vi "calculate_frequency.vi"(8 "error in (no error)":errorcluster, 10 "array with duplicates removed":string[](array[string]), 11 "String data spreadsheet":string) -> (0 "error out":errorcluster, 1 "Array":i32[](array[numeric]), 2 "Frequency of numbers":string[][](array[string]), 3 "Cluster":cluster{i32[], i32[]})   [LabVIEW 2020]
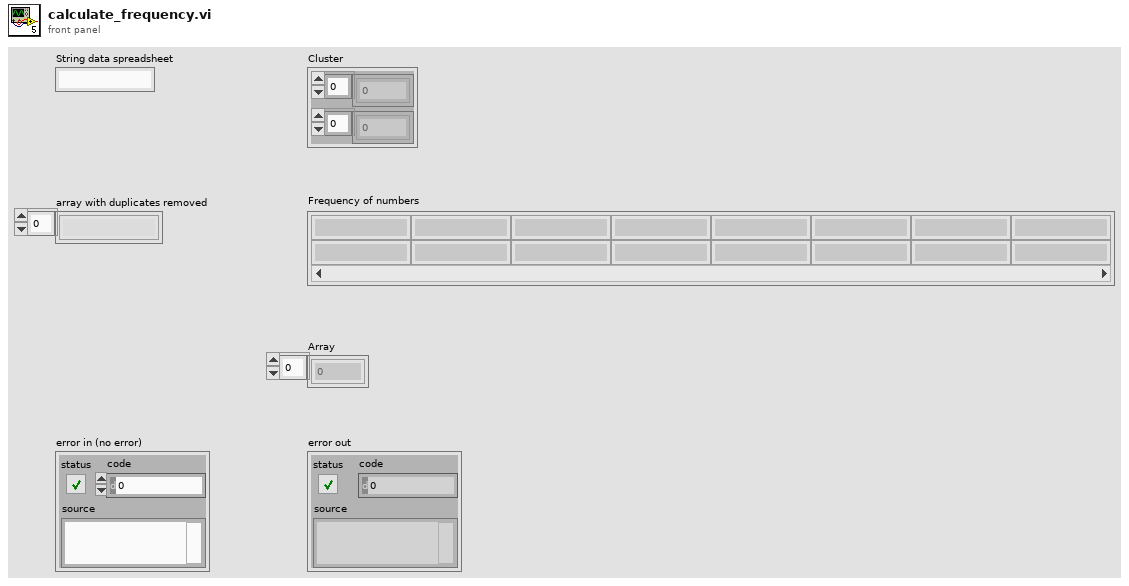
[diagram p1: front panel]
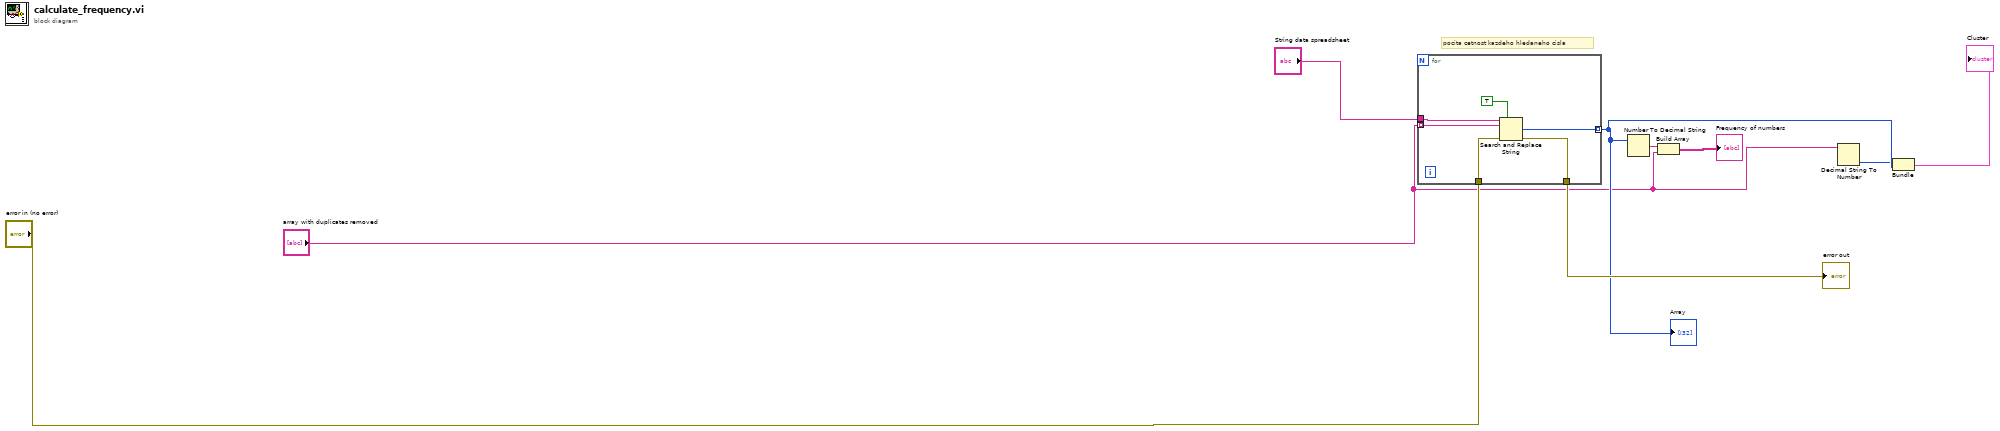
[diagram p0: block diagram]
diagram:
  # "pocita cetnost kazdeho hledaneho cisla"
  n1 = for {
    tunnel: "array with duplicates removed" -> [w13] mode=indexing
    tunnel: [w14] -> w7 mode=indexing
    tunnel: "String data spreadsheet" -> [w12]
    tunnel: "error in (no error)" -> [w11]
    tunnel: [w10] -> w9
    n2 = Search and Replace String(replace all?=TRUE ("replace all? (F)"), input string=w12, search string=w13, error in=w11) -> (number of replacements=w14:i32, error out=w10:errorcluster)  [unwired: 4 in, 2 out]
  }
  "error out" <- w9
  "Array" <- w7
  n3 = Number To Decimal String(number=w7) -> (decimal integer string=w2:string[])  [unwired: 1 in]
  n4 = Build Array(w2, "array with duplicates removed") -> (→"Frequency of numbers":string[][])
  n5 = Decimal String To Number(string="array with duplicates removed") -> (number=w3:i32[])  [unwired: 2 in, 1 out]
  n6 = Bundle(w3, w7) -> (→"Cluster":cluster{i32[], i32[]})  [unwired: 1 in]
